vi "RSZVB Get Time Gate Shape.vi"(8 "error in (no error)":errorcluster {"code" format="%.0x"}, 10 "Channel (Trace) (1)":i32=1, 11 "VISA session":refnum<visa-resource-name>) -> (0 "error out":errorcluster {"code" format="%.0x"}, 2 "Time Gate Shape":i32, 3 "dup VISA session":refnum<visa-resource-name>)   [LabVIEW 2011]
doc: "This VI returns the time gate applied to the time domain transform.\n\nRemote-control command(s):\nCALCulate<Ch/Tr>:FILTer[:GATE]:TIME:SHAPe?"
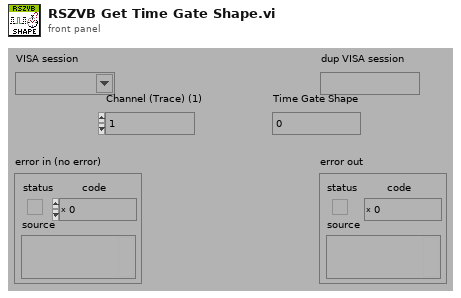
[diagram p1: front panel]
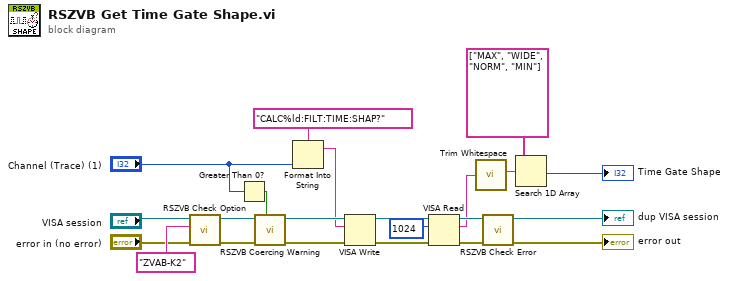
[diagram p0: block diagram]
diagram:
  n1 = call "RSZVB Check Option.vi"("error in (no error)"="error in (no error)", "Options"="ZVAB-K2", "VISA session"="VISA session") -> ("error out"=w4:errorcluster, "dup VISA session"=w3:refnum<visa-resource-name>)  [unwired: 7 in]
  n2 = Greater Than 0?(x="Channel (Trace) (1)") -> (x > 0?=w13:bool)
  n3 = call "RSZVB Coercing Warning.vi"("In Range?"=w13, "error in (no error)"=w4, "VISA session"=w3) -> ("error out"=w20:errorcluster, "dup VISA session"=w21:refnum<visa-resource-name>)  [unwired: 7 in]
  n4 = Format Into String(format string="CALC%ld:FILT:TIME:SHAP?", "Channel (Trace) (1)") -> (resulting string=w19:string)  [unwired: 2 in, 1 out]
  n5 = VISA Write(VISA resource name=w21, write buffer=w19, error in (no error)=w20) -> (VISA resource name out=w15:refnum<visa-resource-name>, error out=w14:errorcluster)  [unwired: 1 out]
  n6 = VISA Read(VISA resource name=w15, byte count=u32 1024 ("byte count (0)"), error in (no error)=w14) -> (VISA resource name out=w17:refnum<visa-resource-name>, read buffer=w10:string, error out=w16:errorcluster)  [unwired: 1 out]
  n7 = call <vilib>:"Trim Whitespace.vi"("string"=w10) -> ("trimmed string"=w12:string)  [unwired: 1 in]
  n8 = call "RSZVB Check Error.vi"("error in (no error)"=w16, "VISA session"=w17) -> ("error out"=→"error out":errorcluster, "dup VISA session"=→"dup VISA session":refnum<visa-resource-name>)  [unwired: 8 in]
  n9 = Search 1D Array(1D array=string[] ["MAX", "WIDE", "NORM", "MIN"] ("array 2"), element=w12) -> (index of element=→"Time Gate Shape":i32)  [unwired: 1 in]
